vi "Monitor-example.vi"(8 "error in (no error)":errorcluster, 11 "Errors in":T1) -> (0 "error out":errorcluster, 3 "Errors out":T1)   [LabVIEW 2013]
uses:
  Errors.lvclass
  Object-reference.ctl
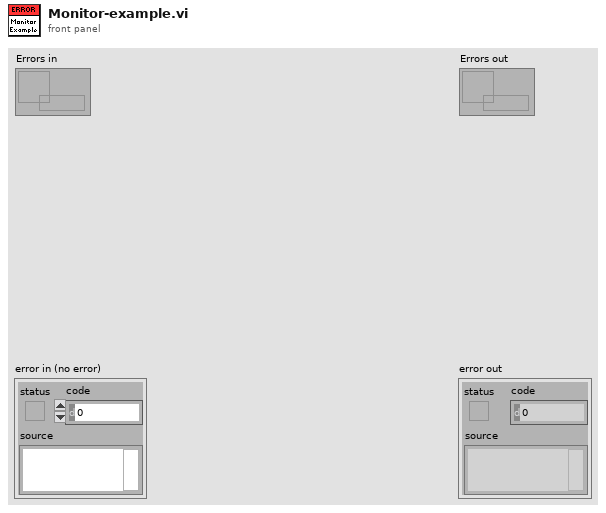
[diagram p1: front panel]
types:
  T1 = typedef "Error-handling.lvlib/Errors.lvclass/Object-reference.ctl" = refnum<data-value>
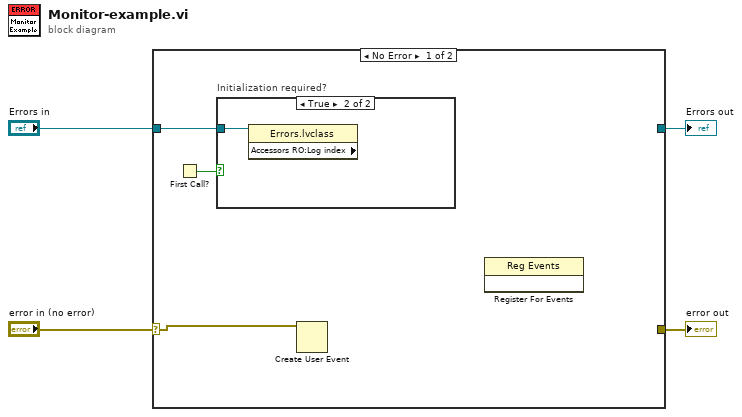
[diagram p0: block diagram]
diagram:
  n1 = case shown="No Error" "error in (no error)" {
    selector: "error in (no error)" -> [w5 w9]
    tunnel: [_ w9] -> w3
    tunnel: [_ w10] -> w1
    tunnel: "Errors in" -> [w6 w10]
    frame No Error {
      n2 = First Call?() -> (First Call?: T/F=w7:bool)
      n3 = case "Initialization required?" shown="True" w7 {
        tunnel: w6 -> [_ w8]
        frame False {
        }
        frame True {
          n4 = property class="Errors.lvclass" props=["Accessors RO:Log index"](reference=w8) -> ()  [unwired: 1 in, 3 out]
        }
      }
      n5 = Create User Event(user event datatype=w5) -> ()  [unwired: 1 in, 2 out]
      n6 = register-events() -> ()  [unwired: 3 in, 2 out]
    }
    frame Error {
    }
  }
  "error out" <- w3
  "Errors out" <- w1
